vi "Write Diagram.vi"(5 "Diagram.lvclass":refnum<class "Diagram.lvclass">, 9 "FlatSequenceFrame in":refnum<class "FlatSequenceFrame.lvclass">) -> (3 "FlatSequenceFrame out":refnum<class "FlatSequenceFrame.lvclass">)   [LabVIEW 2014, in "Raspberry Pi Compatible Compiler for LabVIEW.lvlib" / "FlatSequenceFrame.lvclass"]
uses:
  FlatSequenceFrame.lvclass
  Diagram/Diagram.lvclass
  FlatSequenceFrame.lvclass/FlatSequenceFrame.ctl
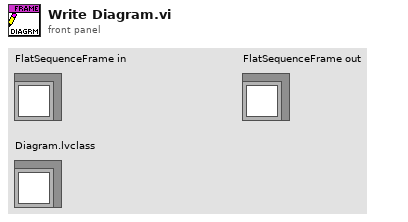
[diagram p1: front panel]
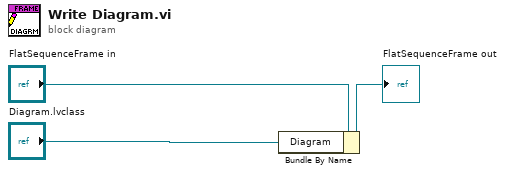
[diagram p0: block diagram]
diagram:
  n1 = Bundle By Name(cluster="FlatSequenceFrame in", "Diagram"="Diagram.lvclass") -> (→"FlatSequenceFrame out":refnum<class "FlatSequenceFrame.lvclass">)
